vi "Operator Input click on choice with pic.vi"(6 "Zoom factor":dbl=0.5 min=0.2 max=3.0 step=0.1, 7 "path to JPEG file":path=path "l:/Programs/Nimbelink/Skywire/Pictures/1002213/pic1.JPG", 8 "error in (no error)":errorcluster, 9 "button2 text":string, 10 "button1 text":string, 11 "Operator text":string) -> (0 "error out":errorcluster, 2 "button2 clicked?":bool, 3 "button1 clicked or space bar hit?":bool)   [LabVIEW 2013]
uses:
  <vilib>/event_ctls.llb/eventvkey.ctl
  <vilib>/picture/picture.llb/Draw True-Color Pixmap.vi
panel:
  out "picture":picture
  in  "button2 clicked":bool caption="button2 clicked?"
  in  "button1 clicked or space bar":bool caption="button1 clicked?"
  out "Message":string
  # "Operator Message"
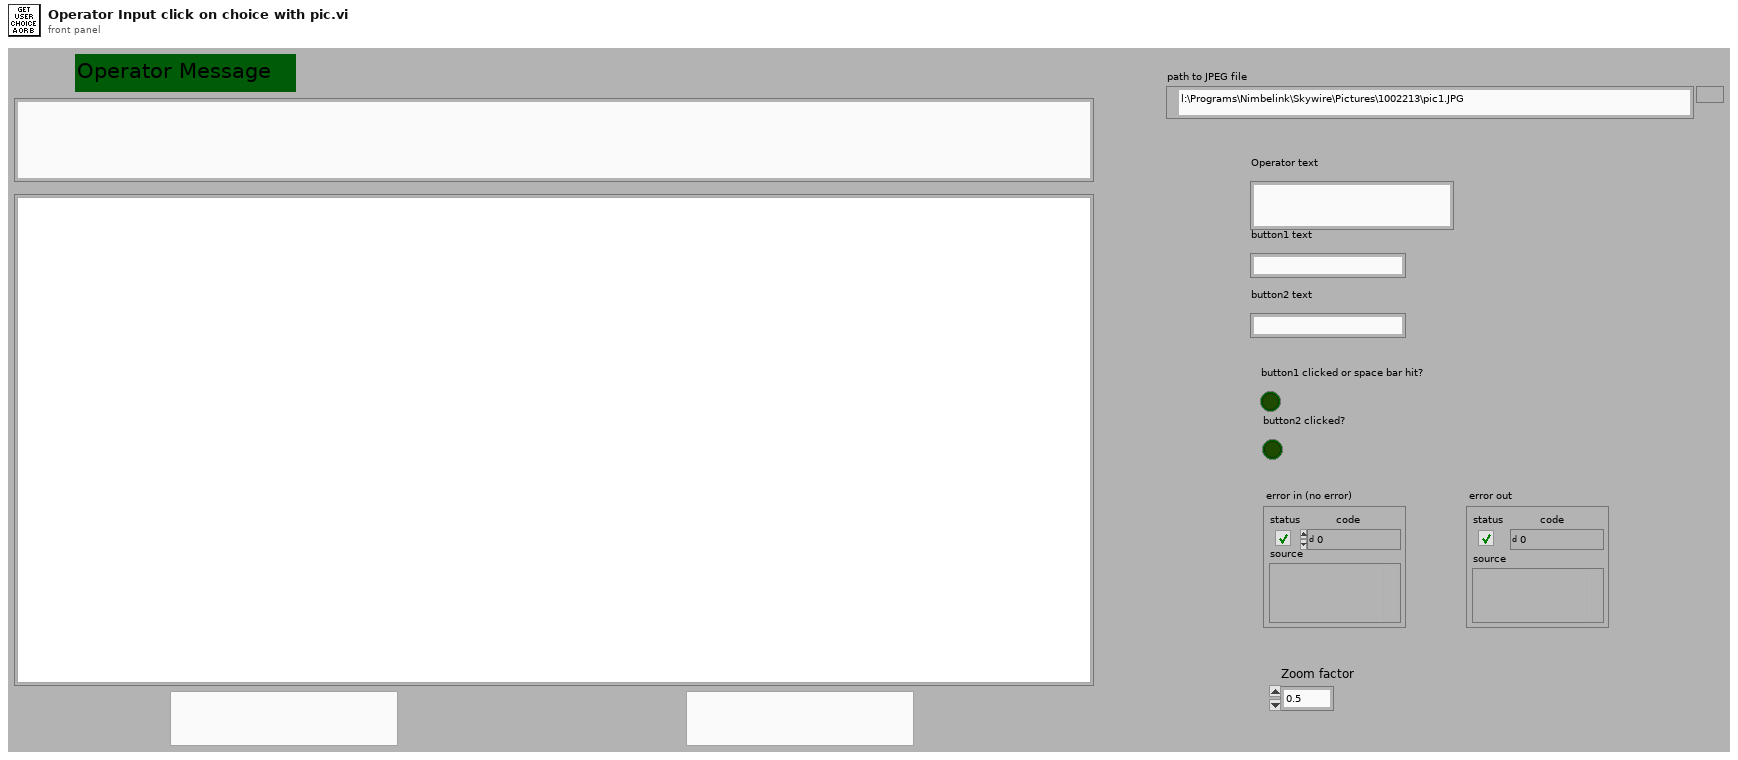
[diagram p1: front panel]
types:
  T1 = typedef "imagedata.ctl" = cluster{"image type":i32, "image depth":i32, "image":u8[], "mask":u8[], "colors":u32[], "Rectangle":cluster{"left":i16, "top":i16, "right":i16, "bottom":i16}}
  T2 = typedef "LVBoundsTypeDef.ctl" = cluster{"Width":u32, "Height":u32}
  T3 = typedef "eventvkey.ctl" = enum16{"ASCII", "Enter", "Return", "Shift", "Ctrl", "Alt", "Cmd", "Opt", "Caps", "NumLock", "Clear", "Break", "Up", "Down", "Left", "Right", "Insert", "Delete", "Home", "End", "PageUp", "PageDown", "Escape", "Help", "Pause", "ScrollLock", "F1", "F2", "F3", "F4", "F5", "F6", "F7", "F8", "F9", "F10", "F11", "F12", "F13", "F14", "F15", "F16", "F17", "F18", "F19", "F20", "F21", "F22", "F23", "F24", "Play", "VolumeUp", "VolumeDown", "Mute", "Two Byte Char"}
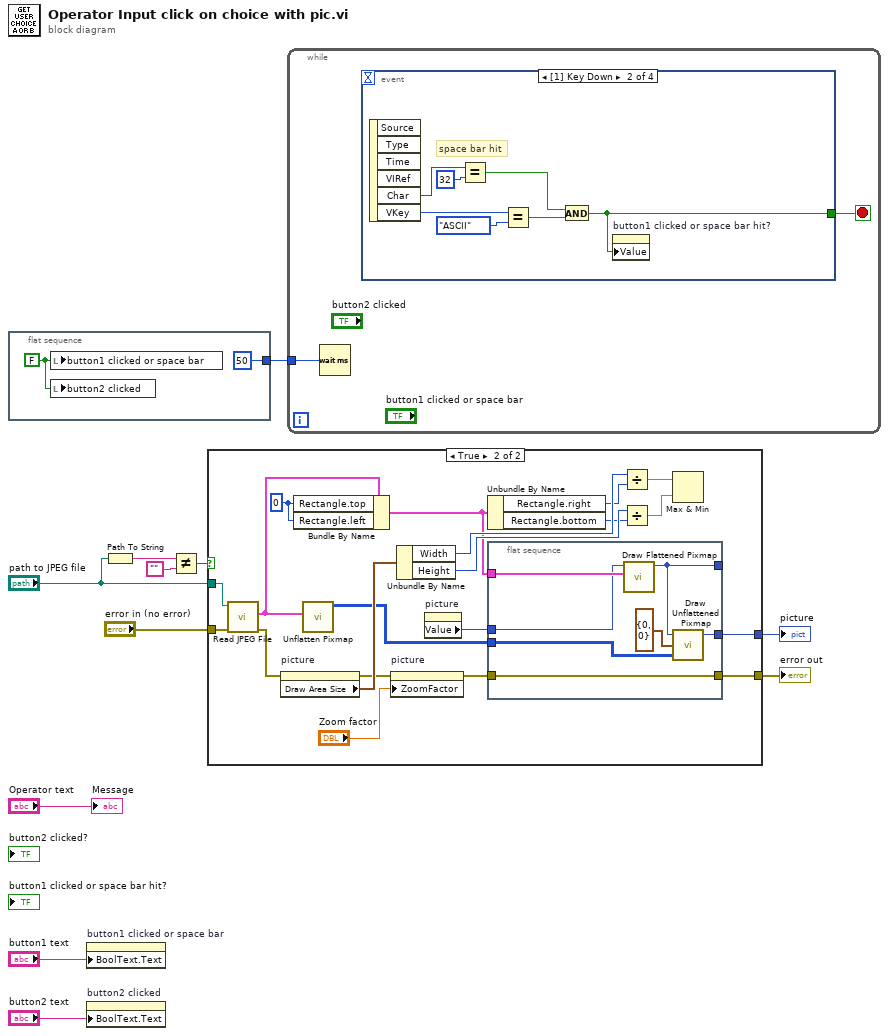
[diagram p0: block diagram]
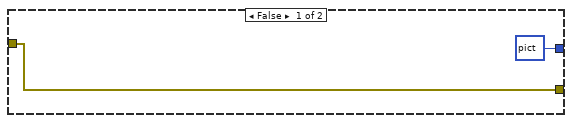
[diagram p2: hidden frame]
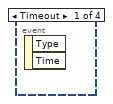
[diagram p3: hidden frame]
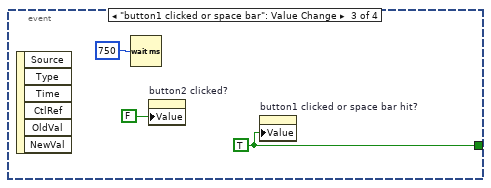
[diagram p4: hidden frame]
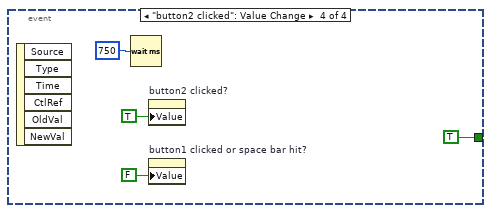
[diagram p5: hidden frame]
diagram:
  n1 = flat-sequence {
    tunnel: [u32 50 ("milliseconds to wait")] -> w11
    frame #0 {
      w12 = FALSE ("button1")
      n2 = local write "button1 clicked or space bar"(w12) -> ()
      n3 = local write "button2 clicked"(w12) -> ()
    }
  }
  n4 = property on="button1 clicked or space bar" class="Bool (strict)"("BoolText.Text"="button1 text") -> ()  [unwired: 2 in, 2 out]
  n5 = property on="button2 clicked" class="Bool (strict)"("BoolText.Text"="button2 text") -> ()  [unwired: 2 in, 2 out]
  n6 = Path To String(path="path to JPEG file") -> (string=w6:string)
  n7 = Not Equal?(x=w6, y="") -> (x != y?=w7:bool)
  n8 = case shown="True" w7 {
    tunnel: "error in (no error)" -> [w15 w28]
    tunnel: "path to JPEG file" -> [_ w23]
    tunnel: [picture data[5B] ("new picture") w17] -> w1
    tunnel: [w15 w24] -> w2
    frame False {
    }
    frame True {
      w20 = i16 0 ("Rectangle.top")
      n9 = call <vilib>:"Read JPEG File.vi"("error in (no error)"=w28, "path to JPEG file"=w23) -> ("error out"=w27:errorcluster, "image data"=w19:T1)  [unwired: 7 in, 1 out]
      n10 = property on="picture" class="Pict"(error in=w27) -> (error out=w26:errorcluster, "Draw Area Size"=w35:T2)  [unwired: 1 in, 1 out]
      n11 = Bundle By Name(cluster=w19, "Rectangle.top"=w20, "Rectangle.left"=w20) -> (w21:T1)
      n12 = call <vilib>:"Unflatten Pixmap.vi"("image data"=w19) -> ("24-bit pixmap"=w18:u32[][])  [unwired: 4 in, 6 out]
      n13 = property on="picture" class="Pict"(error in=w26, "ZoomFactor"="Zoom factor") -> (error out=w25:errorcluster)  [unwired: 1 in, 1 out]
      n14 = Unbundle By Name(w35) -> ("Width"=w32:u32, "Height"=w30:u32)
      n15 = property on="picture" class="Pict"() -> ("Value"=w22:picture)  [unwired: 2 in, 2 out]
      n16 = Unbundle By Name(w21) -> ("Rectangle.right"=w31:i16, "Rectangle.bottom"=w29:i16)
      n17 = flat-sequence {
        tunnel: [w39] -> _
        tunnel: w21 -> [w42]
        tunnel: w25 -> [w41]
        tunnel: [w41] -> w24
        tunnel: w22 -> [w40]
        tunnel: w18 -> [w37]
        tunnel: [w36] -> w17
        frame #0 {
          n18 = call <vilib>:"Draw Flattened Pixmap.vi"("image data"=w42, "picture"=w40) -> ("new picture"=w39:picture)  [unwired: 7 in]
          n19 = call-poly <vilib>:"Draw Unflattened Pixmap.vi"("picture"=w39, "top left point(0, 0)"=cluster{"x":i16, "y":i16} {"x"=0, "y"=0}, "data (RGB format)"=w37) -> ("new picture"=w36:picture)  [unwired: 6 in]
        }
      }
      n20 = Divide(x=w32, y=w31) -> (x/y=w34:dbl)
      n21 = Divide(x=w30, y=w29) -> (x/y=w33:dbl)
      n22 = Max & Min(x=w34, y=w33) -> ()  [unwired: 2 out]
    }
  }
  "error out" <- w2
  "picture" <- w1
  n23 = while {
    tunnel: w11 -> [w44]
    stop <- w43 stop-if-true
    n24 = Wait (ms)(milliseconds to wait=w44) -> ()  [unwired: 1 out]
    n25 = event shown="[1] Key Down" {
      selector: _ -> [_ _ _ _]
      dyn-events: _ -> [_ _ _ _]
      timeout: _ -> [_ _ _ _]
      tunnel: [_ w45 w54 TRUE] -> w43
      event Timeout {
        n26 = event-data() -> ()  [unwired: 1 in, 2 out]
      }
      event Key Down {
        # "space bar hit"
        n27 = event-data() -> ("Char"=w51:i16, "VKey"=w48:T3)  [unwired: 1 in, 4 out]
        n28 = Equal?(x=w51, y=i16 32) -> (x = y?=w47:bool)
        n29 = Equal?(x=w48, y=eventvkey."ASCII" ("VKey")) -> (x = y?=w46:bool)
        n30 = And(x=w47, y=w46) -> (x .and. y?=w45:bool)
        n31 = property on="button1 clicked or space bar hit?" class="Bool (strict)"("Value"=w45) -> ()  [unwired: 2 in, 2 out]
      }
      event "button1 clicked or space bar": Value Change {
        w54 = TRUE
        n32 = event-data() -> ()  [unwired: 1 in, 6 out]
        n33 = Wait (ms)(milliseconds to wait=u32 750) -> ()  [unwired: 1 out]
        n34 = property on="button2 clicked?" class="Bool (strict)"("Value"=FALSE ("button2 clicked?")) -> ()  [unwired: 2 in, 2 out]
        n35 = property on="button1 clicked or space bar hit?" class="Bool (strict)"("Value"=w54) -> ()  [unwired: 2 in, 2 out]
      }
      event "button2 clicked": Value Change {
        n36 = event-data() -> ()  [unwired: 1 in, 6 out]
        n37 = Wait (ms)(milliseconds to wait=u32 750) -> ()  [unwired: 1 out]
        n38 = property on="button2 clicked?" class="Bool (strict)"("Value"=TRUE ("button2 clicked?")) -> ()  [unwired: 2 in, 2 out]
        n39 = property on="button1 clicked or space bar hit?" class="Bool (strict)"("Value"=FALSE ("button1 clicked?")) -> ()  [unwired: 2 in, 2 out]
      }
    }
  }
  "Message" <- "Operator text"
